vi "send rel move to sample stage.vi"(8 "error in (no error)":errorcluster, 11 "Autofocus in":refnum<class "Autofocus.lvclass">) -> (0 "error out":errorcluster, 3 "Autofocus out":refnum<class "Autofocus.lvclass">)   [LabVIEW 2012]
uses:
  <vilib>/Distrio/Murmex/Message/Message.lvclass
  <vilib>/Distrio/Murmex/Murmex/Murmex.lvclass
  <vilib>/Distrio/Murmex/GenericMessage/GenericMessage.lvclass
  Autofocus.lvclass
  <vilib>/Distrio/Murmex/StartMessage/StartMessage.lvclass
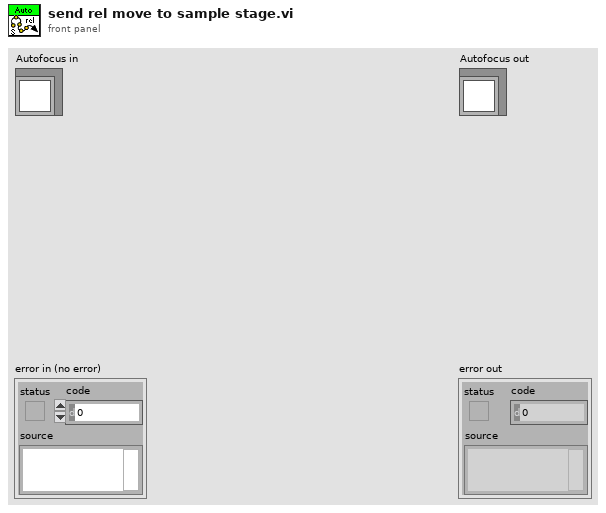
[diagram p1: front panel]
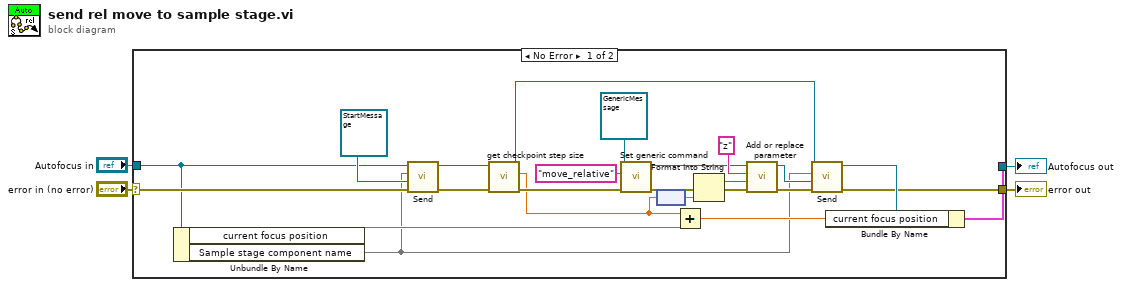
[diagram p0: block diagram]
diagram:
  n1 = case shown="No Error" "error in (no error)" {
    selector: "error in (no error)" -> [w11 w30]
    tunnel: [w17 w30] -> w3
    tunnel: [w16 w29] -> w1
    tunnel: "Autofocus in" -> [w5 w29]
    frame No Error {
      n2 = Unbundle By Name(w5) -> ("current focus position"=w12, "Sample stage component name"=w6)
      n3 = call <vilib>:"Send.vi"("error in (no error)"=w11, "Message"=refnum<class "StartMessage.lvclass"> refnum ("Message in"), "recipient"=w6, "Murmex in"=w5) -> ("error out"=w9:errorcluster, "Murmex out"=w10:refnum<class "Autofocus.lvclass">)  [unwired: 6 in]
      n4 = call-dynamic "get checkpoint step size.vi"("error in (no error)"=w9, "Autofocus in"=w10) -> ("error out"=w15:errorcluster, "checkpoint stepsize"=w13:dbl[unit], "Autofocus out"=w8:refnum<class "Autofocus.lvclass">)  [unwired: 7 in]
      n5 = call <vilib>:"Set generic command.vi"("error in (no error)"=w15, "generic command"="move_relative" ("command string"), "GenericMessage in"=refnum<class "GenericMessage.lvclass"> refnum ("Murmex.lvlib:GenericMessage")) -> ("error out"=w21:errorcluster, "GenericMessage out"=w20:refnum<class "GenericMessage.lvclass">)  [unwired: 7 in]
      n6 = node(w13) -> (w14:dbl)
      n7 = Add(x=w13, y=w12) -> (x+y=w18:dbl[unit])
      n8 = Format Into String(error in=w21, w14) -> (resulting string=w25:string, error out=w24:errorcluster)  [unwired: 2 in]
      n9 = call <vilib>:"Add or replace parameter.vi"("error in (no error)"=w24, "value"=w25, "name"="z", "Message in"=w20) -> ("error out"=w27:errorcluster, "Message out"=w28:refnum<class "GenericMessage.lvclass">)  [unwired: 6 in]
      n10 = call <vilib>:"Send.vi"("error in (no error)"=w27, "Message"=w28, "recipient"=w6, "Murmex in"=w8) -> ("error out"=w17:errorcluster, "Murmex out"=w19:refnum<class "Autofocus.lvclass">)  [unwired: 6 in]
      n11 = Bundle By Name(cluster=w19, "current focus position"=w18) -> (w16:cluster{})
    }
    frame Error {
    }
  }
  "error out" <- w3
  "Autofocus out" <- w1
